vi "Write Updates.vi"(11 "DaqControl in":T1) -> (3 "DaqControl out":T1)   [LabVIEW 2020, in "VolatusDaq.lvlib" / "DaqControl.lvclass"]
uses:
  DaqControl.lvclass
  Loop Data.ctl
  Volatus/Event API/EventAPI.lvclass
  Volatus/DataHandlerAPI/DataHandlerAPI.lvclass
  Sequence Action.ctl
  Seq Action Type.ctl
  Value Update.ctl
  Seq Cmd.ctl
  Seq Cmd Type.ctl
  Signal Type.ctl
  Volatus/DataHandlerAPI/DataHandlerAPI.lvclass/DataHandlerAPI.ctl
  Volatus/DataHandler Messages/New Data Msg/New Data Msg.lvclass/New Data Msg.ctl
  <vilib>/ActorFramework/Message Enqueuer/Message Enqueuer.lvclass/Message Enqueuer.ctl
  Volatus/Event API/EventAPI.lvclass/EventAPI.ctl
  Volatus/EventHandler Messages/Handle Event Msg/Handle Event Msg.lvclass/Handle Event Msg.ctl
  <vilib>/DAQmx/write.llb/DAQmx Write (Analog 1D DBL NChan 1Samp).vi
  <vilib>/DAQmx/write.llb/DAQmx Write (Digital 1D Bool NChan 1Samp 1Line).vi
  lv-vecto/Vecto/Bool to Double.vi
  Volatus/Event API/Report Event.vi
  Volatus/DataHandler Messages/New Data Msg/Send New Data.vi
  Volatus/EventHandler Messages/Handle Event Msg/Send Handle Event.vi
  <vilib>/ActorFramework/Message Enqueuer/Enqueue.vi
  Volatus/DataHandler Messages/New Data Msg/New Data Msg.lvclass
  C:/Program Files (x86)/National Instruments/LabVIEW 2020/vi.lib/ActorFramework/Message/Message.lvclass
  Volatus/EventHandler Messages/Handle Event Msg/Handle Event Msg.lvclass
  <vilib>/DAQmx/miscellaneous.llb/DAQmx Fill In Error Info.vi
  <vilib>/ActorFramework/Message Priority Queue/Priority Enqueue.vi
  DaqControl.lvclass/DaqControl.ctl
  VolatusDaq.lvlib
  Sequence.ctl
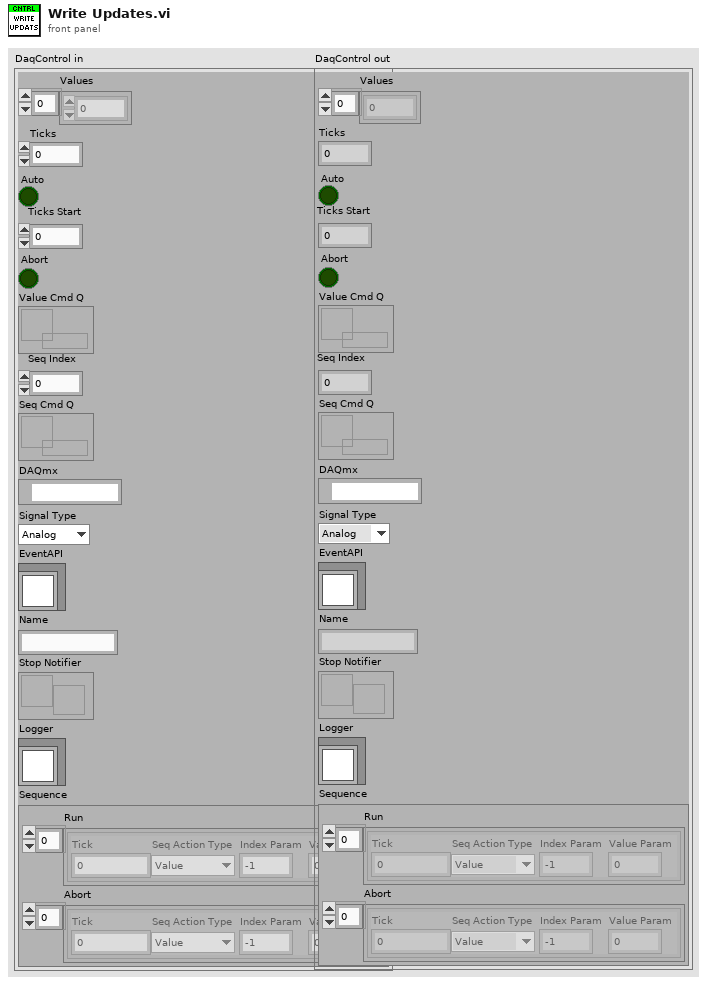
[diagram p1: front panel]
types:
  T1 = typedef "VolatusDaq.lvlib/DaqControl.lvclass/Loop Data.ctl" = cluster{"Values":dbl[], "Ticks":u32, "Auto":bool, "Ticks Start":u32, "Abort":bool, "Value Cmd Q":refnum<queue>, "Seq Index":i32, "Seq Cmd Q":refnum<queue>, "DAQmx":refnum<k21>, "Signal Type":T2, "EventAPI":refnum<class "EventAPI.lvclass">, "Name":string, "Stop Notifier":refnum<notifier>, "Logger":refnum<class "DataHandlerAPI.lvclass">, "Sequence":T3}
  T2 = typedef "VolatusDaq.lvlib/Signal Type.ctl" = enum16{"Analog", "Digital"}
  T3 = typedef "VolatusDaq.lvlib/Sequence.ctl" = cluster{"Run":T4[], "Abort":T4[]}
  T4 = typedef "VolatusDaq.lvlib/Sequence Action.ctl" = cluster{"Tick":u32, "Seq Action Type":T5, "Index Param":i32, "Value Param":dbl}
  T5 = typedef "VolatusDaq.lvlib/Seq Action Type.ctl" = enum16{"Value", "Stop"}
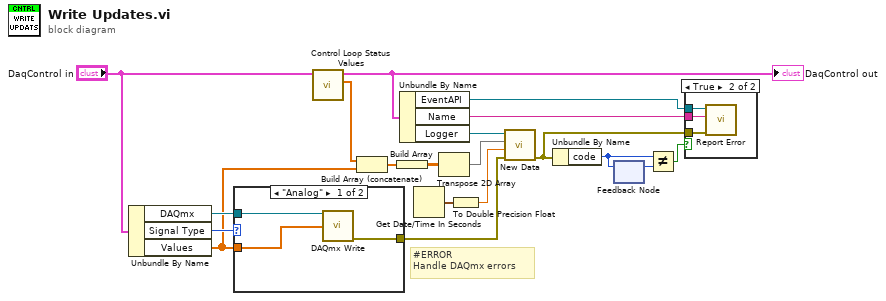
[diagram p0: block diagram]
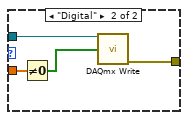
[diagram p3: hidden frame]
diagram:
  # "#ERROR\nHandle DAQmx errors"
  n1 = Unbundle By Name("DaqControl in") -> ("DAQmx"=w18:refnum<k21>, "Signal Type"=w19:T2, "Values"=w16:dbl[])
  n2 = case shown="\"Analog\"" w19 {
    tunnel: w16 -> [w21 w26]
    tunnel: w18 -> [w22 w25]
    tunnel: [w20 w23] -> w4
    frame "Analog" {
      n3 = call-poly <vilib>:"DAQmx Write.vi"("task/channels in"=w22, "data"=w21) -> ("error out"=w20:errorcluster)  [unwired: 11 in, 2 out]
    }
    frame "Digital" {
      n4 = Not Equal To 0?(x=w26) -> (x != 0?=w24:bool[])
      n5 = call-poly <vilib>:"DAQmx Write.vi"("task/channels in"=w25, "data"=w24) -> ("error out"=w23:errorcluster)  [unwired: 11 in, 2 out]
    }
  }
  n6 = call "Control Loop Status Values.vi"("Loop Data in"="DaqControl in") -> ("Status Values"=w13:dbl[], "Loop Data"=w15:T1)  [unwired: 9 in]
  "DaqControl out" <- w15
  n7 = Build Array (concatenate)(w13, w16) -> (w14:dbl[])
  n8 = Build Array(w14) -> (w9:dbl[][])
  n9 = Unbundle By Name(w15) -> ("EventAPI"=w12:refnum<class "EventAPI.lvclass">, "Name"=w11:string, "Logger"=w8:refnum<class "DataHandlerAPI.lvclass">)
  n10 = Get Date/Time In Seconds() -> (seconds since 1Jan1904=w6:timestamp)
  n11 = Transpose 2D Array(2D array=w9) -> (transposed array=w7:dbl[][])
  n12 = To Double Precision Float(number=w6) -> (double precision float=w5:dbl)
  n13 = call "New Data.vi"("error in (no error)"=w4, "t0"=w5, "Data"=w7, "DataHandlerAPI in"=w8) -> ("error out"=w1:errorcluster)  [unwired: 6 in, 1 out]
  n14 = Unbundle By Name(w1) -> ("code"=w3:i32)
  n15 = feedback-in #1(w3) -> ()
  n16 = feedback #1() -> (w2:i32)  [unwired: 1 in]
  n17 = Not Equal?(x=w3, y=w2) -> (x != y?=w10:bool)
  n18 = case shown="True" w10 {
    tunnel: w12 -> [_ w29]
    tunnel: w11 -> [_ w28]
    tunnel: w1 -> [_ w27]
    frame False {
    }
    frame True {
      n19 = call "Report Error.vi"("error in (no error)"=w27, "Context"=w28, "Event API in"=w29) -> ()  [unwired: 7 in, 2 out]
    }
  }
